vi "Untitled 2.vi"() -> ()   [LabVIEW 2010]
uses:
  Control 1.ctl
panel:
  out "suma":dbl
  in  "init":bool
  in  "передати":bool
  in  "stop":bool
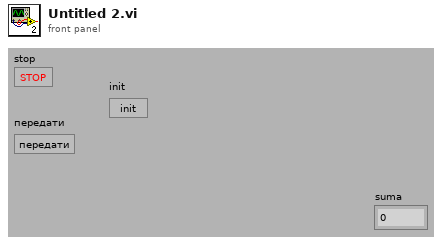
[diagram p1: front panel]
types:
  T1 = typedef "Control 1.ctl" = enum16{"старт", "init", "стоп"}
  T2 = enum32{"Invalid", "Standard", "Closed", "Hidden", "Minimized", "Maximized"}
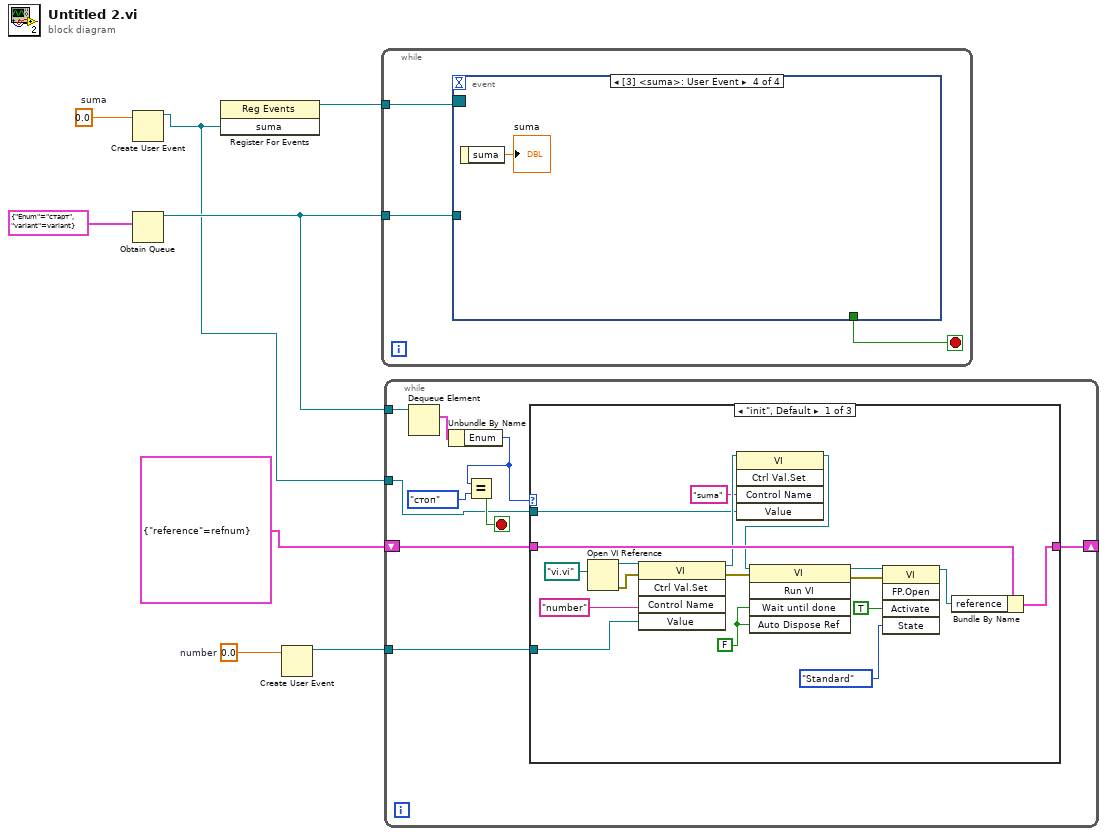
[diagram p0: block diagram]
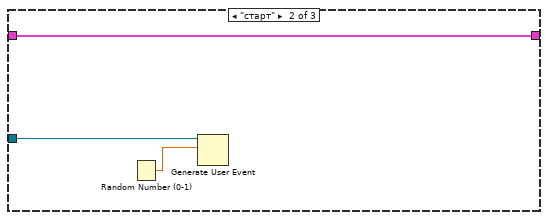
[diagram p2: hidden frame]
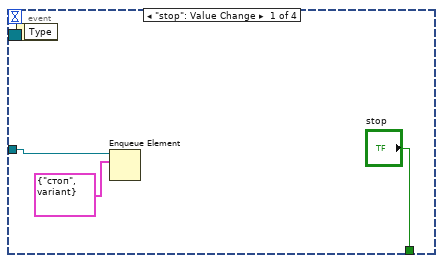
[diagram p4: hidden frame]
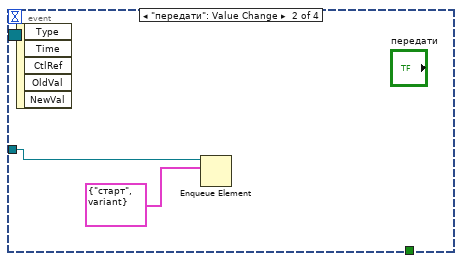
[diagram p5: hidden frame]
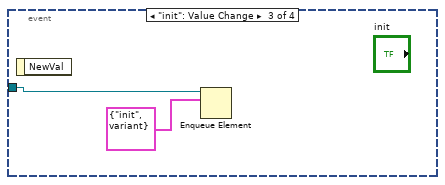
[diagram p6: hidden frame]
diagram:
  w2 = 0.0  # suma
  w5 = 0.0  # number
  n1 = Create User Event(user event datatype=w2) -> (user event=w1:refnum<user-event>)  [unwired: 1 in, 1 out]
  n2 = Obtain Queue(element data type=cluster{"Enum":T1, "variant":variant} {"Enum"=enum."старт", "variant"=variant}) -> (queue out=w7:refnum<queue>)  [unwired: 4 in, 2 out]
  n3 = register-events(w1) -> (reference out=w3:refnum<event-registration>)  [unwired: 2 in, 1 out]
  n4 = Create User Event(user event datatype=w5) -> (user event=w4:refnum<user-event>)  [unwired: 1 in, 1 out]
  n5 = while {
    tunnel: w7 -> [w10]
    tunnel: w3 -> [w9]
    stop <- w11 stop-if-true
    n6 = event shown="[3] <suma>: User Event" {
      selector: w9 -> [_ _ _ _]
      dyn-events: _ -> [_ _ _ _]
      timeout: _ -> [_ _ _ _]
      tunnel: ["stop" _ _ _] -> w11
      tunnel: w10 -> [w13 w16 w18 _]
      event "stop": Value Change {
        n7 = event-data() -> ()  [unwired: 1 in, 1 out]
        n8 = Enqueue Element(queue=w13, element=cluster{"Enum":T1, "variant":variant} {"Enum"=enum."стоп", "variant"=variant}) -> ()  [unwired: 2 in, 3 out]
      }
      event "передати": Value Change {
        n9 = event-data() -> ()  [unwired: 1 in, 5 out]
        n10 = Enqueue Element(queue=w16, element=cluster{"Enum":T1, "variant":variant} {"Enum"=enum."старт", "variant"=variant}) -> ()  [unwired: 2 in, 3 out]
      }
      event "init": Value Change {
        n11 = event-data() -> ()  [unwired: 1 in, 1 out]
        n12 = Enqueue Element(queue=w18, element=cluster{"Enum":T1, "variant":variant} {"Enum"=enum."init", "variant"=variant}) -> ()  [unwired: 2 in, 3 out]
      }
      event User Event {
        n13 = event-data() -> ("suma"=→"suma":dbl)  [unwired: 1 in]
      }
    }
  }
  n14 = while {
    tunnel: w7 -> [w28]
    shift-right: [w22] -> _
    shift-left: cluster{"reference":refnum<vi>} {"reference"=refnum} -> [w23]
    tunnel: w4 -> [w21]
    tunnel: w1 -> [w20]
    stop <- w24 stop-if-true
    n15 = Dequeue Element(queue=w28) -> (element=w27:cluster{"Enum":T1, "variant":variant})  [unwired: 2 in, 3 out]
    n16 = Unbundle By Name(w27) -> ("Enum"=w25:T1)
    n17 = Equal?(x=w25, y=Control_1."стоп" ("Enum")) -> (x = y?=w24:bool)
    n18 = case shown="\"init\", Default" w25 {
      tunnel: w23 -> [w40 w49 w50]
      tunnel: [w39 w49 w50] -> w22
      tunnel: w21 -> [w38 w48 _]
      tunnel: w20 -> [w29 _ _]
      frame "init", Default {
        w45 = FALSE ("Wait Until Done")
        n19 = Open VI Reference(vi path=path "vi.vi") -> (vi reference=w35:refnum<vi>, error out=w34:errorcluster)  [unwired: 5 in]
        n20 = invoke class="VI" method="Ctrl Val.Set"(reference=w35, error in=w34, "Control Name"="number", "Value"=w38) -> (reference out=w32:refnum<vi>, error out=w33:errorcluster)  [unwired: 1 in, 3 out]
        n21 = invoke class="VI" method="Ctrl Val.Set"(reference=w32, "Control Name"="suma", "Value"=w29) -> (reference out=w31:refnum<vi>)  [unwired: 2 in, 4 out]
        n22 = invoke class="VI" method="Run VI"(reference=w31, error in=w33, "Wait until done"=w45, "Auto Dispose Ref"=w45) -> (reference out=w44:refnum<vi>, error out=w41:errorcluster)  [unwired: 1 in, 3 out]
        n23 = invoke class="VI" method="FP.Open"(reference=w44, error in=w41, "Activate"=TRUE ("Activate?"), "State"=T2."Standard") -> (reference out=w36:refnum<vi>)  [unwired: 1 in, 4 out]
        n24 = Bundle By Name(cluster=w40, "reference"=w36) -> (w39:cluster{"reference":refnum<vi>})
      }
      frame "старт" {
        n25 = Random Number (0-1)() -> (number: 0 to 1=w47:dbl)
        n26 = Generate User Event(user event=w48, event data cluster=w47) -> ()  [unwired: 1 in, 2 out]
      }
      frame "стоп" {
      }
    }
  }
